vi "Write Tag.vi"(8 "error in (no error)":errorcluster, 10 "Tag":string, 11 "MenuItem in":refnum<class "MGI_MenuItem.lvclass">) -> (0 "error out":errorcluster, 3 "MenuItem out":refnum<class "MGI_MenuItem.lvclass">)   [LabVIEW 2016, in "MGI_MenuItem.lvclass"]
doc: "This can be used to identify the menu item even after the text has been changed. The tag is used when building the full tag. If a Tag is not defined when the menu is being initialized, then the current Name of the MenuItem is used.\n\nThe menu tag cannot be changed after the menu has been initialized.\n\nAuthored by Derek E. Trepanier\nsupport@mooregoodideas.com\nwww.mooregoodideas.com\n\nCopyright (c) 2012, Moore Good Ideas, Inc.\n\nAll rights reserved.\n\nRedistribution and use in source and binary forms, with or without modification, are permitted provided that the following conditions are met:\n\n * Redistributions of source code must retain the above copyright notice, this list of conditions and the following disclaimer.\n * Redistributions in binary form must reproduce the above copyright notice, this list of conditions and the following disclaimer in the documentation and/or other materials provided with the distribution.\n * Neither the name of Moore Good Ideas, Inc. nor the names of its contributors may be used to endorse or promote products derived from this software without specific prior written permission.\n\nTHIS SOFTWARE IS PROVIDED BY THE COPYRIGHT HOLDERS AND CONTRIBUTORS \"AS IS\" AND ANY EXPRESS OR IMPLIED WARRANTIES, INCLUDING, BUT NOT LIMITED TO, THE IMPLIED WARRANTIES OF MERCHANTABILITY AND FITNESS FOR A PARTICULAR PURPOSE ARE DISCLAIMED. IN NO EVENT SHALL THE COPYRIGHT OWNER OR CONTRIBUTORS BE LIABLE FOR ANY DIRECT, INDIRECT, INCIDENTAL, SPECIAL, EXEMPLARY, OR CONSEQUENTIAL DAMAGES (INCLUDING, BUT NOT LIMITED TO, PROCUREMENT OF SUBSTITUTE GOODS OR SERVICES; LOSS OF USE, DATA, OR PROFITS; OR BUSINESS INTERRUPTION) HOWEVER CAUSED AND ON ANY THEORY OF LIABILITY, WHETHER IN CONTRACT, STRICT LIABILITY, OR TORT (INCLUDING NEGLIGENCE OR OTHERWISE) ARISING IN ANY WAY OUT OF THE USE OF THIS SOFTWARE, EVEN IF ADVISED OF THE POSSIBILITY OF SUCH DAMAGE."
uses:
  <userlib>/_MGI/Menu Building/MenuItem/MGI_MenuItem.lvclass
  <userlib>/_MGI/Menu Building/MenuItem/MGI_MenuItem.lvclass/MGI_MenuItem.ctl
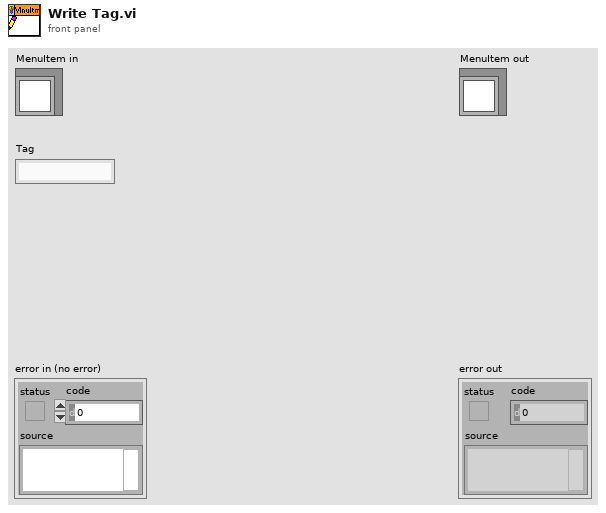
[diagram p1: front panel]
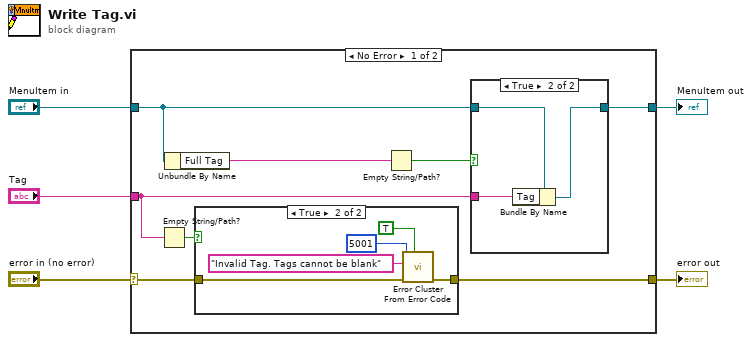
[diagram p0: block diagram]
diagram:
  n1 = case shown="No Error" "error in (no error)" {
    selector: "error in (no error)" -> [w6 w24]
    tunnel: [w7 w24] -> w4
    tunnel: [w13 w25] -> w2
    tunnel: "MenuItem in" -> [w12 w25]
    tunnel: "Tag" -> [w9 _]
    frame No Error {
      n2 = Empty String/Path?(string/path=w9) -> (empty?=w8:bool)
      n3 = Unbundle By Name(w12) -> ("Full Tag"=w11:string)
      n4 = case shown="True" w8 {
        tunnel: [w14 w18] -> w7
        tunnel: w6 -> [w14 w19]
        frame False {
        }
        frame True {
          n5 = call <vilib>:"Error Cluster From Error Code.vi"("show call chain? (False)"=TRUE, "error in (no error)"=w19, "error message (\"\")"="Invalid Tag. Tags cannot be blank" ("error message (\"\")"), "error code (0)"=5001) -> ("error out"=w18:errorcluster)  [unwired: 5 in]
        }
      }
      n6 = Empty String/Path?(string/path=w11) -> (empty?=w10:bool)
      n7 = case shown="True" w10 {
        tunnel: [w20 w23] -> w13
        tunnel: w12 -> [w20 w22]
        tunnel: w9 -> [_ w21]
        frame False {
          # "The menu has already been initialized. Changing the tag now will mess up the clicking logic."
        }
        frame True {
          n8 = Bundle By Name(cluster=w22, "Tag"=w21) -> (w23:refnum<class "MGI_MenuItem.lvclass">)
        }
      }
    }
    frame Error {
    }
  }
  "error out" <- w4
  "MenuItem out" <- w2
